vi "Epsilon Compare.vi"(8 "Epsilon":dbl, 10 "Value2":dbl, 11 "Value1":dbl) -> (3 "Boolean":bool)   [LabVIEW 2013]
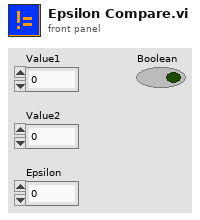
[diagram p1: front panel]
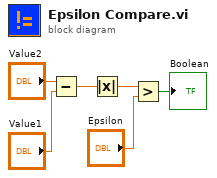
[diagram p0: block diagram]
diagram:
  n1 = Subtract(x="Value2", y="Value1") -> (x-y=w2:dbl)
  n2 = Absolute Value(x=w2) -> (abs(x)=w3:dbl)
  n3 = Greater?(x=w3, y="Epsilon") -> (0:→"Boolean":bool)
